vi "Update.vi"(8 "error in (no error)":errorcluster, 10 "Message in":refnum<class "UpdateMessage.lvclass">, 11 "focus in":refnum<class "focus.lvclass">) -> (0 "error out":errorcluster, 3 "focus out":refnum<class "focus.lvclass">)   [LabVIEW 2012, in "focus.lvclass"]
doc: "The update method processes the command 'update'. \n\nThe command 'update' is used for receiving new values to be set to the private data of the class. This could be seen as a public set method for setting new parameters to the private class data."
uses:
  focus.lvclass
  <vilib>/Distrio/Murmex/UpdateMessage/UpdateMessage.lvclass
  focus.lvclass/focus.ctl
  <vilib>/Distrio/Murmex/Murmex/Murmex.lvclass
panel:
  # "This method is called when the UPDATE\ntrigger is sent. \n\nOverride this method when your component needs to\nrespond to this trigger. \n\nCall parent for proper implementation"
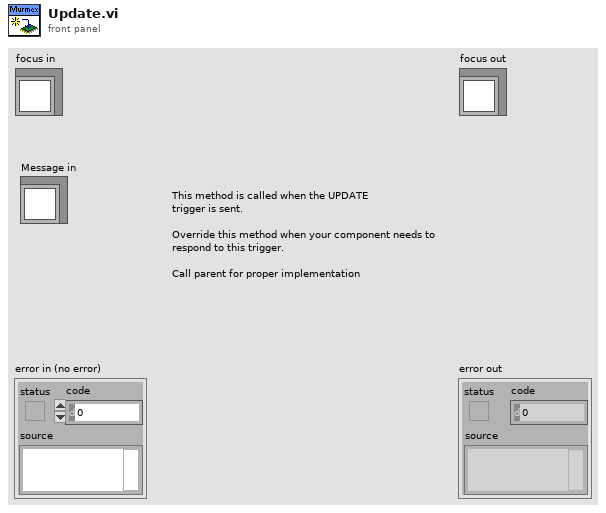
[diagram p1: front panel]
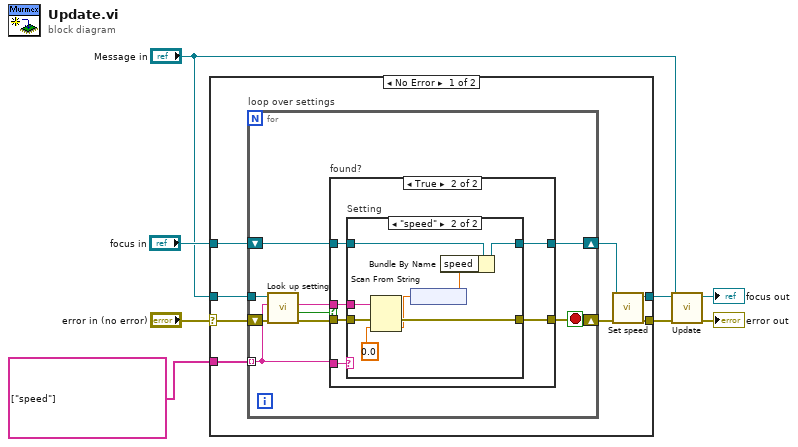
[diagram p0: block diagram]
diagram:
  n1 = case shown="No Error" "error in (no error)" {
    selector: "error in (no error)" -> [w15 w44]
    tunnel: "focus in" -> [w13 w45]
    tunnel: "Message in" -> [w14 _]
    tunnel: string[] ["speed"] ("key chains") -> [w16 _]
    tunnel: [w11 w44] -> w2
    tunnel: [w9 w45] -> w1
    frame No Error {
      n2 = for "loop over settings" {
        tunnel: w16 -> [w23] mode=indexing
        tunnel: w14 -> [w24]
        shift-right: [w17] -> w12
        shift-left: w15 -> [w25]
        shift-right: [w18] -> w10
        shift-left: w13 -> [w19]
        stop <- w17 stop-if-true
        n3 = call <vilib>:"Look up setting.vi"("error in (no error)"=w25, "tag name"=w23, "UpdateMessage in"=w24) -> ("error out"=w22:errorcluster, "found?"=w21:bool, "value"=w20:string)  [unwired: 5 in, 1 out]
        n4 = case "found?" shown="True" w21 {
          tunnel: w19 -> [w27 w31]
          tunnel: w20 -> [_ w32]
          tunnel: w22 -> [w26 w30]
          tunnel: w23 -> [_ w33]
          tunnel: [w27 w29] -> w18
          tunnel: [w26 w28] -> w17
          frame False {
          }
          frame True {
            n5 = case "Setting" shown="\"speed\"" w33 {
              tunnel: w32 -> [_ w39]
              tunnel: w31 -> [w35 w41]
              tunnel: w30 -> [w34 w43]
              tunnel: [w35 w40] -> w29
              tunnel: [w34 w42] -> w28
              frame Default {
              }
              frame "speed" {
                n6 = Scan From String(input string=w39, error in=w43, default 1=0.0 ("Settings_cluster.Power")) -> (error out=w42:errorcluster, output 1=w38:dbl)  [unwired: 2 in, 2 out]
                n7 = node(w38) -> (w36:dbl[unit])
                n8 = Bundle By Name(cluster=w41, "speed"=w36) -> (w40:refnum<class "focus.lvclass">)
              }
            }
          }
        }
      }
      n9 = call-dynamic "Set speed.vi"("error in (no error)"=w12, "focus in"=w10) -> ("error out"=w11:errorcluster, "focus out"=w9:refnum<class "focus.lvclass">)  [unwired: 8 in]
    }
    frame Error {
    }
  }
  n10 = call-parent "Update.vi"("error in (no error)"=w2, "Message in"="Message in", "Murmex in"=w1) -> ("error out"=→"error out":errorcluster, "Murmex out"=→"focus out":refnum<class "focus.lvclass">)  [unwired: 7 in]
